vi "check_signal_chopper_state.vi"(7 "parity?":bool, 10 "chopper":bool[](array[boolean]), 11 "data":dbl[][](array[numeric])) -> (2 "chopper out":bool[](array[boolean]), 3 "data out":dbl[][](array[numeric]))   [LabVIEW 2019]
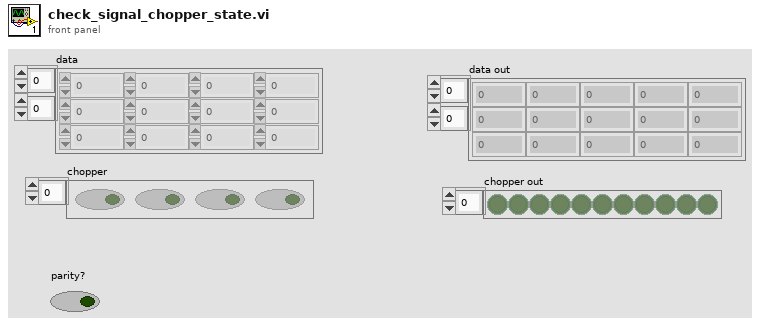
[diagram p1: front panel]
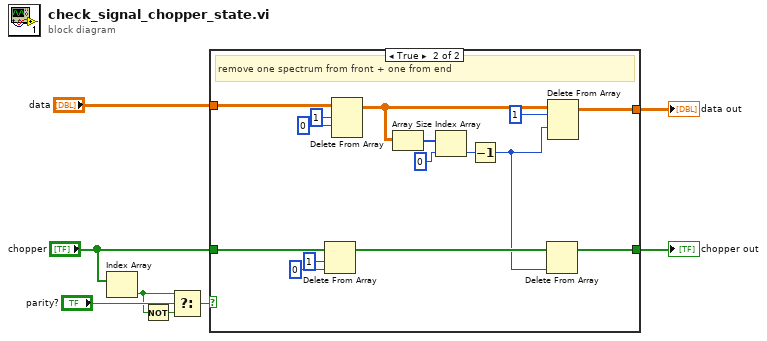
[diagram p0: block diagram]
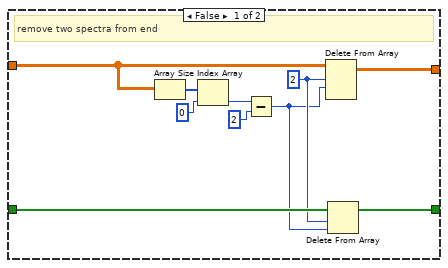
[diagram p2: hidden frame]
diagram:
  n1 = Index Array(array="chopper") -> (element=w3:bool)  [unwired: 1 in]
  n2 = Not(x=w3) -> (.not. x?=w2:bool)
  n3 = Select(t=w3, s="parity?", f=w2) -> (s? t:f=w5:bool)
  n4 = case shown="True" w5 {
    tunnel: "data" -> [w15 w27]
    tunnel: [w16 w31] -> w8
    tunnel: "chopper" -> [w12 w23]
    tunnel: [w9 w19] -> w7
    frame False {
      w11 = 2 ("length")
      # "remove two spectra from end"
      n5 = Array Size(array=w15) -> (size(s)=w18:i32[])
      n6 = Index Array(array=w18, index=0) -> (element=w14:i32)
      n7 = Subtract(x=w14, y=2) -> (x-y=w10:i32)
      n8 = Delete From Array(array=w15, length=w11, index (row)=w10) -> (array with subset deleted=w16:dbl[][])  [unwired: 1 in, 1 out]
      n9 = Delete From Array(array=w12, length=w11, index=w10) -> (array with subset deleted=w9:bool[])  [unwired: 1 out]
    }
    frame True {
      # "remove one spectrum from front + one from end"
      n10 = Delete From Array(array=w23, length=1, index=0 ("index (row)")) -> (array with subset deleted=w22:bool[])  [unwired: 1 out]
      n11 = Delete From Array(array=w27, length=1, index (row)=0) -> (array with subset deleted=w26:dbl[][])  [unwired: 1 in, 1 out]
      n12 = Array Size(array=w26) -> (size(s)=w30:i32[])
      n13 = Index Array(array=w30, index=0) -> (element=w28:i32)
      n14 = Decrement(x=w28) -> (x-1=w20:i32)
      n15 = Delete From Array(array=w22, index=w20) -> (array with subset deleted=w19:bool[])  [unwired: 1 in, 1 out]
      n16 = Delete From Array(array=w26, length=1, index (row)=w20) -> (array with subset deleted=w31:dbl[][])  [unwired: 1 in, 1 out]
    }
  }
  "data out" <- w8
  "chopper out" <- w7
